vi "Read Color Cluster.vi"(8 "error in (no error)":errorcluster, 9 "Active Plot":i32, 11 "3D Contour in":refnum<class "3D Contour.lvclass">) -> (0 "error out":errorcluster, 2 "Color Ramp Cluster":T1={"Color Ramp Style"=enum."None", "Color Ramp Array"=[16711934, 393471, 57855, 4390754, 16449346, 16744722, 16711680], "Color Ramp Index"=[45, 91, 133, 175, 219, 255], "Interpolate?"=FALSE, "Logarithm?"=FALSE}, 3 "3D Contour out":refnum<class "3D Contour.lvclass">)   [LabVIEW 2017, in "3D Contour.lvclass"]
uses:
  <vilib>/Math Plots/3D Math Plots/3D Contour/3D Contour/3D Contour.lvclass
  <vilib>/Math Plots/3D Math Plots/3D Plot/3D Plot/Typedef/Color Ramp Cluster.ctl
  <vilib>/Math Plots/3D Math Plots/3D Contour/3D Contour/3D Contour.lvclass/3D Contour.ctl
  <vilib>/Math Plots/3D Math Plots/3D Plot/3D Plot/3D Plot.lvclass
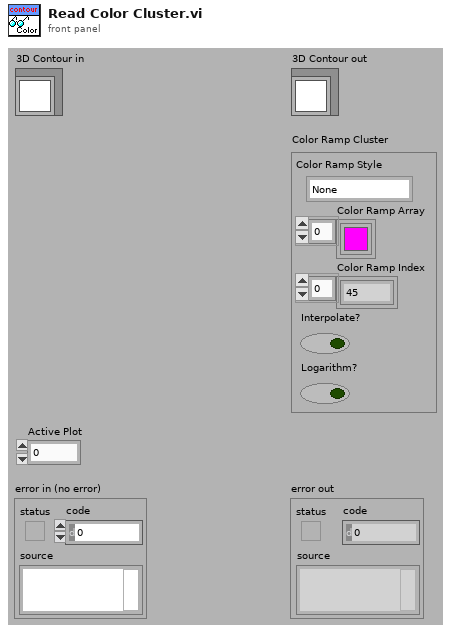
[diagram p1: front panel]
types:
  T1 = typedef "3D Plot.lvclass/Color Ramp Cluster.ctl" = cluster{"Color Ramp Style":enum16{"None", "Shaded", "Color spectrum", "Grey scale", "Custom"}, "Color Ramp Array":u32[], "Color Ramp Index":i32[], "Interpolate?":bool, "Logarithm?":bool}
  T2 = typedef "3D Contour.lvclass/3D Contour Property Array.ctl" = T3[]
  T3 = typedef "3D Contour.lvclass/3D Contour Property.ctl" = cluster{"General Property":cluster{"Plot Name":string, "Coordinate System":enum16{"Cartesian", "Cylindrical", "Spherical"}, "Opacity":sgl}, "Projection Property":cluster{"Draw XY":bool, "Draw YZ":bool, "Draw XZ":bool}, "Plot Property":cluster{"Line Style":T4, "Line Width":sgl, "Line Color":u32, "Antialiasing":bool, "Color Ramp Cluster":T1}, "Contour Property":cluster{"Contour Type":enum16{"Contour", "Contour with surface"}, "Axis Basis":enum16{"X-Axis", "Y-Axis", "Z-Axis"}, "Level List":sgl[], "Level Mode":enum16{"Levels", "Interval", "Level List"}, "Levels":u16, "Interval":sgl}}
  T4 = typedef "3D Plot.lvclass/Line Type.ctl" = enum16{"None", "Solid", "Dash", "Dot", "Dash Dot"}
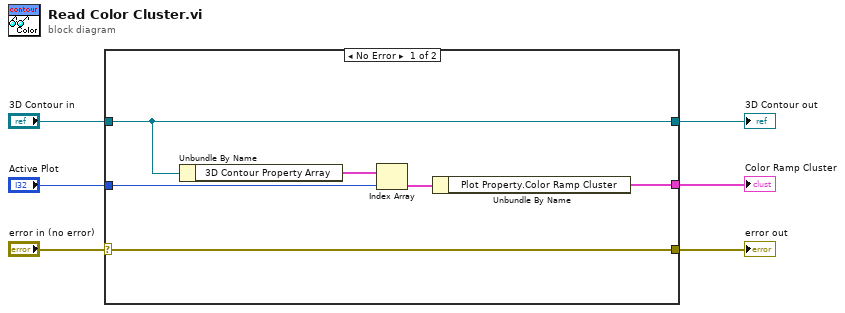
[diagram p0: block diagram]
diagram:
  n1 = case shown="No Error" "error in (no error)" {
    selector: "error in (no error)" -> [w12 w14]
    tunnel: "3D Contour in" -> [w11 w13]
    tunnel: [w11 w13] -> w5
    tunnel: [w12 w14] -> w1
    tunnel: "Active Plot" -> [w9 _]
    tunnel: [w7 _] -> w2
    frame No Error {
      n2 = Unbundle By Name(w11) -> ("3D Contour Property Array"=w10:T2)
      n3 = Index Array(array=w10, index=w9) -> (element=w8:T3)
      n4 = Unbundle By Name(w8) -> ("Plot Property.Color Ramp Cluster"=w7:T1)
    }
    frame Error {
    }
  }
  "error out" <- w1
  "3D Contour out" <- w5
  "Color Ramp Cluster" <- w2
